vi "testFalse.vi"(8 "error in (no error)":errorcluster) -> (0 "error out":errorcluster)   [LabVIEW 2019, in "AssertionTest.lvlib" / "AssertTrue.lvlib"]
uses:
  AssertTrue.lvlib
  Assertion/Assertion.lvlib
  AssertionTest.lvlib
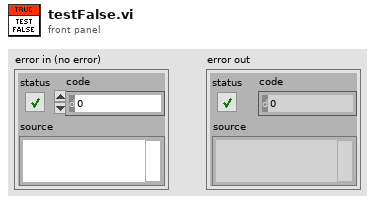
[diagram p1: front panel]
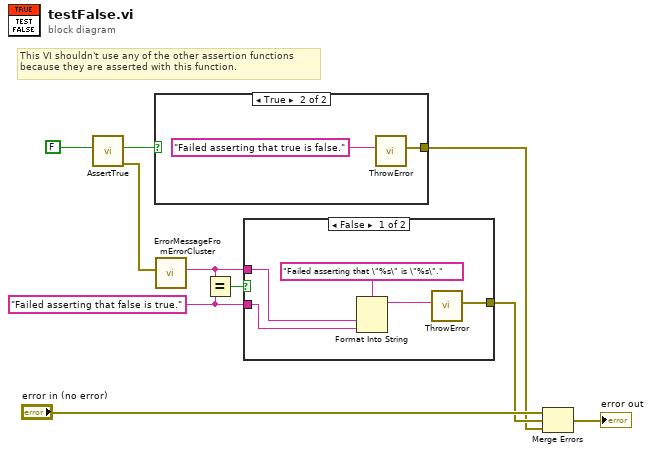
[diagram p0: block diagram]
diagram:
  w7 = "Failed asserting that false is true." ("y")
  # "This VI shouldn't use any of the other assertion functions\nbecause they are asserted with this function."
  n1 = call "AssertTrue.vi"("Condition"=FALSE) -> ("error out"=w6:errorcluster, "Result"=w9:bool)  [unwired: 9 in]
  n2 = case shown="True" w9 {
    tunnel: [_ w11] -> w1
    frame False {
    }
    frame True {
      n3 = call "ThrowError.vi"("Error Message"="Failed asserting that true is false." ("message")) -> ("error out"=w11:errorcluster)  [unwired: 10 in]
    }
  }
  n4 = call "ErrorMessageFromErrorCluster.vi"("Error"=w6) -> ("Error Message"=w5:string)  [unwired: 10 in]
  n5 = Equal?(x=w5, y=w7) -> (x = y?=w8:bool)
  n6 = case shown="False" w8 {
    tunnel: w5 -> [w16 _]
    tunnel: w7 -> [w15 _]
    tunnel: [w13 _] -> w2
    frame False {
      n7 = Format Into String(format string="Failed asserting that \"%s\" is \"%s\".", w16, w15) -> (resulting string=w14:string)  [unwired: 2 in, 1 out]
      n8 = call "ThrowError.vi"("Error Message"=w14) -> ("error out"=w13:errorcluster)  [unwired: 10 in]
    }
    frame True {
    }
  }
  n9 = Merge Errors("error in (no error)", w2, w1) -> (→"error out":errorcluster)
